vi "Decorator.vi"(10 "Actor":refnum<class "Actor.lvclass">, 11 "Developer Utilities in":refnum<class "Developer Utilities.lvclass">) -> (3 "Developer Utilities out":refnum<class "Developer Utilities.lvclass">)   [LabVIEW 2020, in "jettl.lvlib" / "Developer Utilities.lvclass"]
uses:
  Developer Utilities.lvclass
  Actor/Actor/Actor.lvclass
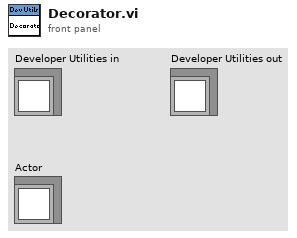
[diagram p1: front panel]
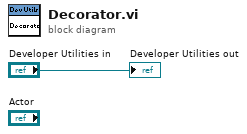
[diagram p0: block diagram]
diagram:
  "Developer Utilities out" <- "Developer Utilities in"
